vi "Decrement Subscribers.vi"(8 "error in (no error)":errorcluster, 11 "CIFChannels in":refnum<class "CIFChannels.lvclass">) -> (0 "error out":errorcluster, 3 "CIFChannels out":refnum<class "CIFChannels.lvclass">)   [LabVIEW 2021, in "CIFChannels.lvclass"]
uses:
  CIFChannels.lvclass
  ChannelCommon/typedef/Channel State.ctl
  CIFChannels.lvclass/CIFChannels.ctl
  ChannelCommon/ChannelCommon.lvlib
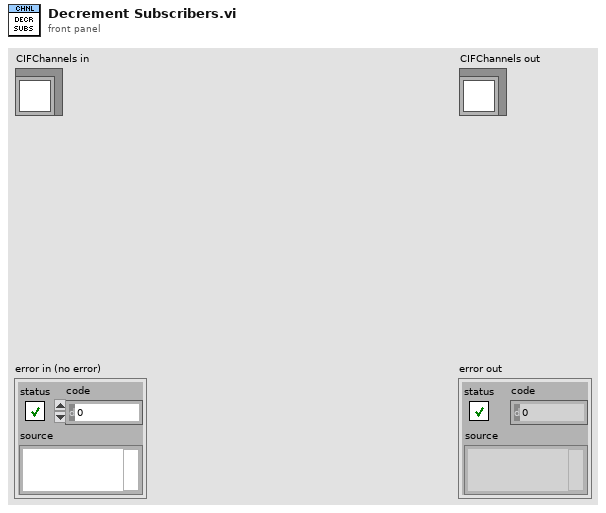
[diagram p1: front panel]
types:
  T1 = typedef "ChannelCommon.lvlib/Channel State.ctl" = enum8{"Creating", "Disconnected", "Connecting", "Connected", "Destroyed"}
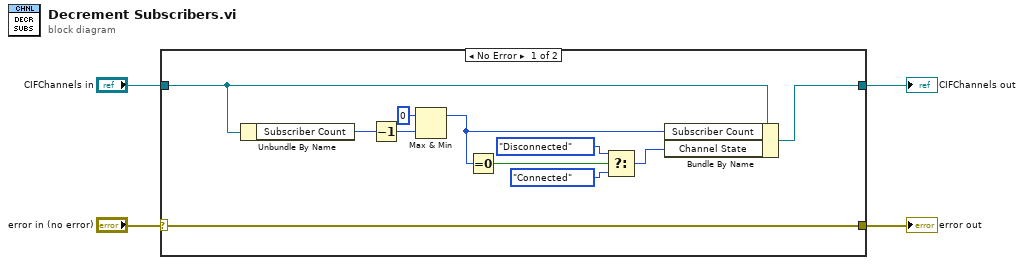
[diagram p0: block diagram]
diagram:
  n1 = case shown="No Error" "error in (no error)" {
    selector: "error in (no error)" -> [w15 w17]
    tunnel: [w15 w17] -> w3
    tunnel: [w13 w16] -> w1
    tunnel: "CIFChannels in" -> [w14 w16]
    frame No Error {
      n2 = Unbundle By Name(w14) -> ("Subscriber Count"=w10:u32)
      n3 = Decrement(x=w10) -> (x-1=w12:u32)
      n4 = Max & Min(x=u32 0, y=w12) -> (max(x,y)=w9:u32)  [unwired: 1 out]
      n5 = Equal To 0?(x=w9) -> (x = 0?=w8:bool)
      n6 = Select(t=Channel_State."Disconnected" ("Channel State"), s=w8, f=Channel_State."Connected" ("Channel State")) -> (s? t:f=w6:T1)
      n7 = Bundle By Name(cluster=w14, "Subscriber Count"=w9, "Channel State"=w6) -> (w13:refnum<class "CIFChannels.lvclass">)
    }
    frame Error {
    }
  }
  "error out" <- w3
  "CIFChannels out" <- w1
